vi "gfitsio-flush-file.vi"(8 "error in (no error)":errorcluster, 11 "gfits refnum":T1) -> (0 "error out":errorcluster, 3 "dup gfits refnum":T1)   [LabVIEW 2022 SP3, in "gfitsio.lvlib"]
doc: "Writes all buffers of the file identified by <B>gfits refnum</B> to disk and updates the directory entry of the file associated with <B>gfits refnum</B>. The file remains open, and refnum remains valid. Data written to a file often resides in a buffer until the buffer fills up or until you close the file. This function forces the cfitsio library and the operating system to write any buffer data to the file."
uses:
  gfitsio.lvlib
  gfitsio-refnum.ctl
  gfitsio.dll
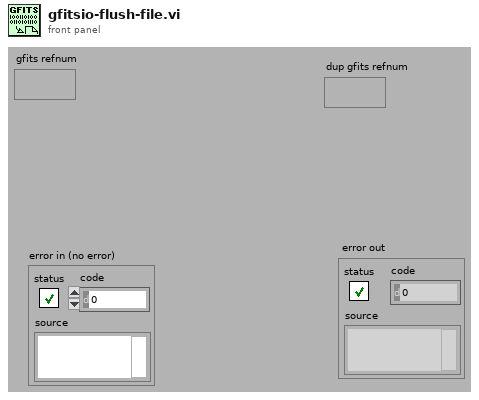
[diagram p1: front panel]
types:
  T1 = typedef "gfitsio.lvlib/gfitsio-refnum.ctl" = refnum<k1>
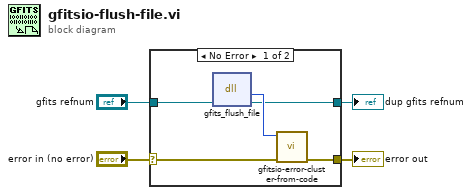
[diagram p0: block diagram]
diagram:
  n1 = case shown="No Error" "error in (no error)" {
    selector: "error in (no error)" -> [w8 w11]
    tunnel: [w7 w11] -> w4
    tunnel: "gfits refnum" -> [w5 w10]
    tunnel: [w6 w10] -> w2
    frame No Error {
      n2 = dll-call lib="C:/Development/rimas/RIMAS/gfitsio/gfitsio.dll" fn="gfits_flush_file"("gfits refnum"=w5) -> (w9:i32, "gfits refnum"=w6:T1)  [unwired: 3 in, 2 out]
      n3 = call "gfitsio-error-cluster-from-code.vi"("error in (no error)"=w8, "error code"=w9) -> ("error out"=w7:errorcluster)  [unwired: 9 out]
    }
    frame Error {
    }
  }
  "error out" <- w4
  "dup gfits refnum" <- w2
